vi "Get Target Type.vi"(11 "FRTS Process in":refnum<class "FRTS Process.lvclass">) -> (2 "Operating System":T1, 3 "FRTS Process out":refnum<class "FRTS Process.lvclass">)   [LabVIEW 2019, in "TimingDRV Engine.lvlib" / "FRTS Process.lvclass"]
uses:
  FRTS Process.lvclass
  <vilib>/NI VeriStand/Custom Device API/Custom Device Target Type.ctl
  FRTS Process.lvclass/FRTS Process.ctl
  <vilib>/NI VeriStand/Custom Device API/Custom Device API.lvlib
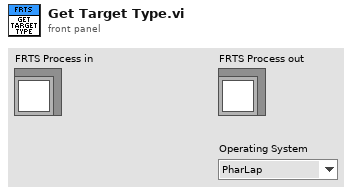
[diagram p1: front panel]
types:
  T1 = typedef "Custom Device API.lvlib/Custom Device Target Type.ctl" = enum16{"PharLap", "VxWorks", "Windows", "Linux_32_ARM", "Linux_x64"}
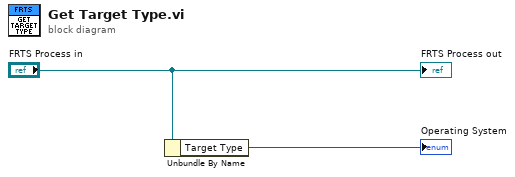
[diagram p0: block diagram]
diagram:
  n1 = Unbundle By Name("FRTS Process in") -> ("Target Type"=→"Operating System":T1)
  "FRTS Process out" <- "FRTS Process in"
